vi "Ephys.vi"() -> ()   [LabVIEW 2010]
uses:
  Electrophysiology/Electrophysiology.lvclass
panel:
  out "FilePath":path
  in  "Recording Channels":refnum<k21>="All4498"
  in  "Stream To":string="localhost"
  out "MSamples":dbl
  in  "Audio":cluster{"Left channel":i32, "Right channel":i32}
  in  "Volume":dbl(slide)=1.0608183551394462e-08 scale=1e-09..1e-05
  in  "Enable Sound":bool
  in  "stop":bool
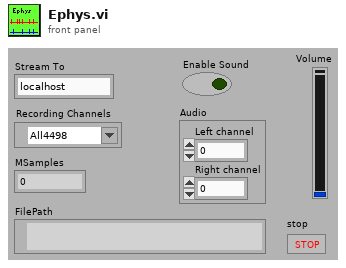
[diagram p1: front panel]
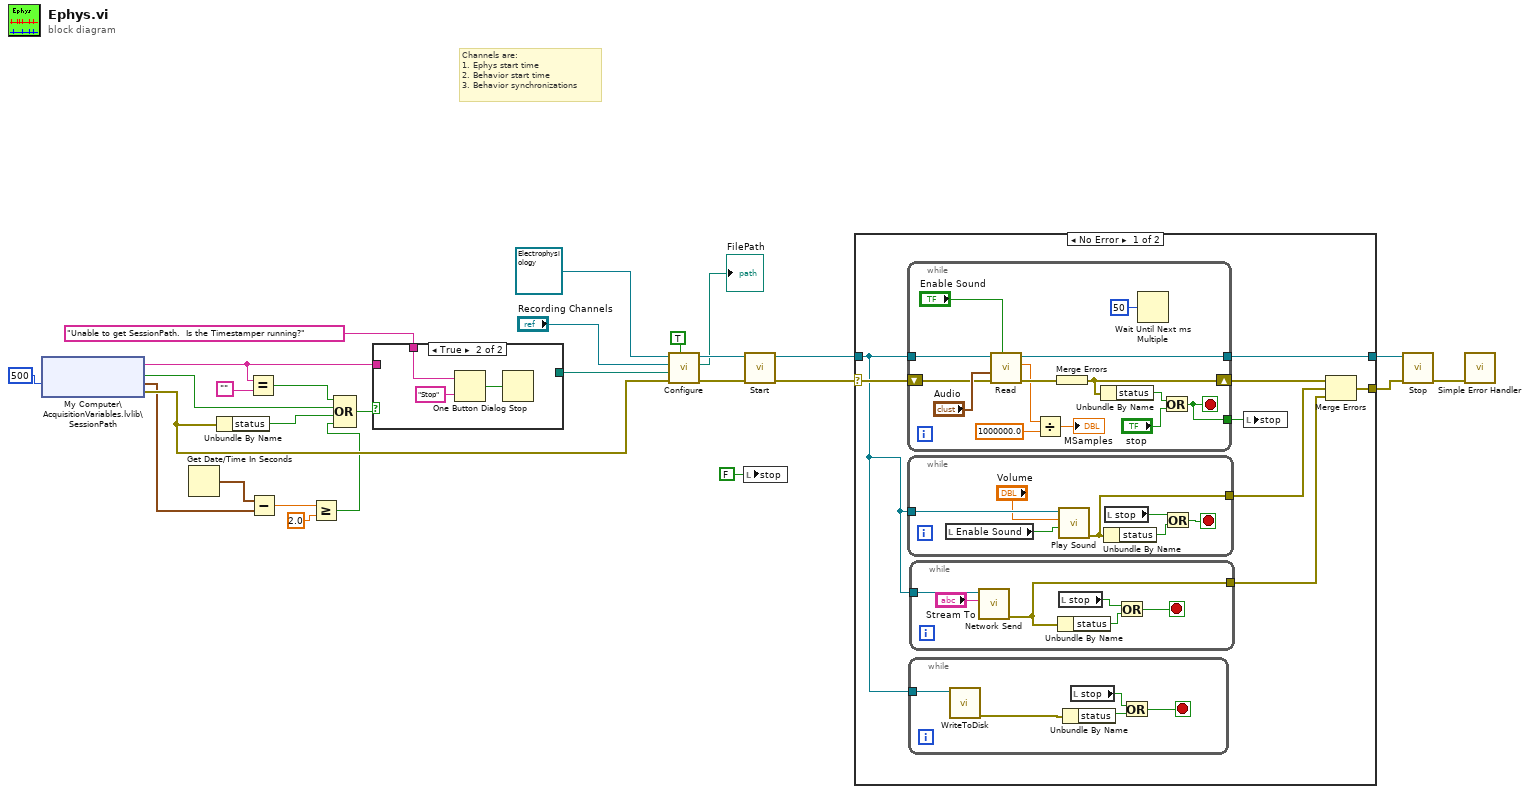
[diagram p0: block diagram]
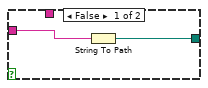
[diagram p2: hidden frame]
diagram:
  # "Channels are:\n1. Ephys start time\n2. Behavior start time\n3. Behavior synchronizations"
  n1 = shared-variable "My Computer\\AcquisitionVariables.lvlib\\SessionPath"(500 ("ms timeout (0)")) -> (w11:string, error out=w9:errorcluster, w15:bool, w4:timestamp)  [unwired: 1 in]
  n2 = Get Date/Time In Seconds() -> (seconds since 1Jan1904=w5:timestamp)
  n3 = Unbundle By Name(w9) -> ("status"=w14:bool)
  n4 = Equal?(x=w11, y="") -> (x = y?=w16:bool)
  n5 = Subtract(x=w5, y=w4) -> (x-y=w3:dbl)
  n6 = Greater Or Equal?(x=w3, y=2.0) -> (x >= y?=w1:bool)
  n7 = Compound Arithmetic op=OR(w16, w15, w14, w1) -> (w13:bool)
  n8 = case shown="True" w13 {
    tunnel: "Unable to get SessionPath.  Is the Timestamper running?" ("message") -> [_ w32]
    tunnel: w11 -> [w29 _]
    tunnel: [w28 _] -> w10
    frame False {
      n9 = String To Path(string=w29) -> (path=w28:path)
    }
    frame True {
      n10 = One Button Dialog(message=w32, button name ("OK")="Stop") -> (true=w31:bool)
      n11 = Stop(stop? (T)=w31) -> ()
    }
  }
  n12 = call-dynamic "Configure.vi"("Enable Sound"=TRUE, "error in (no error)"=w9, "recording path"=w10, "Recording Channels"="Recording Channels", "Electrophysiology in"=refnum<class "Electrophysiology.lvclass"> refnum ("Electrophysiology.lvclass")) -> ("error out"=w26:errorcluster, "FilePath"=→"FilePath":path, "Electrophysiology out"=w27:refnum<class "Electrophysiology.lvclass">)  [unwired: 4 in]
  n13 = local write "stop"(FALSE ("stop")) -> ()
  n14 = call-dynamic "Start.vi"("error in (no error)"=w26, "Electrophysiology in"=w27) -> ("error out"=w23:errorcluster, "Electrophysiology out"=w25:refnum<class "Electrophysiology.lvclass">)  [unwired: 8 in]
  n15 = case shown="No Error" w23 {
    selector: w23 -> [w34 w73]
    tunnel: w25 -> [w33 w74]
    tunnel: [w40 w74] -> w24
    tunnel: [w35 w73] -> w19
    frame No Error {
      n16 = while {
        tunnel: w33 -> [w72]
        tunnel: [w71] -> w40
        tunnel: [w61] -> w39
        shift-right: [w62] -> w38
        shift-left: w34 -> [w60]
        stop <- w61 stop-if-true
        n17 = call-dynamic "Read.vi"("Enable Sound"="Enable Sound", "error in (no error)"=w60, "Audio Channels"="Audio", "Electrophysiology in"=w72) -> ("error out"=w70:errorcluster, "Samples"=w65:dbl, "Electrophysiology out"=w71:refnum<class "Electrophysiology.lvclass">)  [unwired: 5 in]
        n18 = Divide(x=w65, y=1000000.0) -> (x/y=→"MSamples":dbl)
        n19 = Merge Errors(w70) -> (w62:errorcluster)
        n20 = Unbundle By Name(w62) -> ("status"=w69:bool)
        n21 = Wait Until Next ms Multiple(millisecond multiple=u32 50) -> ()  [unwired: 1 out]
        n22 = Or(x=w69, y="stop") -> (x .or. y?=w61:bool)
      }
      n23 = while {
        tunnel: w33 -> [w53]
        tunnel: [w47] -> w37
        stop <- w50 stop-if-true
        n24 = local read "Enable Sound"() -> (w48:bool)
        n25 = call-dynamic "Play Sound.vi"("Enable Sound"=w48, "Volume"="Volume", "Electrophysiology in"=w53) -> ("error out"=w47:errorcluster)  [unwired: 7 in, 1 out]
        n26 = Unbundle By Name(w47) -> ("status"=w51:bool)
        n27 = local read "stop"() -> (w52:bool)
        n28 = Or(x=w52, y=w51) -> (x .or. y?=w50:bool)
      }
      n29 = while {
        tunnel: w33 -> [w58]
        stop <- w54 stop-if-true
        n30 = call "WriteToDisk.vi"("Electrophysiology.lvclass"=w58) -> ("error out"=w57:errorcluster)  [unwired: 8 in, 2 out]
        n31 = Unbundle By Name(w57) -> ("status"=w56:bool)
        n32 = local read "stop"() -> (w55:bool)
        n33 = Or(x=w55, y=w56) -> (x .or. y?=w54:bool)
      }
      n34 = while {
        tunnel: w33 -> [w46]
        tunnel: [w41] -> w36
        stop <- w43 stop-if-true
        n35 = call-dynamic "Network Send.vi"("Target IP Address"="Stream To", "Electrophysiology in"=w46) -> ("error out"=w41:errorcluster)  [unwired: 8 in, 1 out]
        n36 = Unbundle By Name(w41) -> ("status"=w44:bool)
        n37 = local read "stop"() -> (w45:bool)
        n38 = Or(x=w45, y=w44) -> (x .or. y?=w43:bool)
      }
      n39 = local write "stop"(w39) -> ()
      n40 = Merge Errors(w38, w37, w36) -> (w35:errorcluster)
    }
    frame Error {
    }
  }
  n41 = call-dynamic "Stop.vi"("error in (no error)"=w19, "Electrophysiology in"=w24) -> ("error out"=w8:errorcluster)  [unwired: 8 in, 1 out]
  n42 = call <vilib>:"Simple Error Handler.vi"("error in (no error)"=w8) -> ()  [unwired: 4 in, 5 out]
